vi "PWM FPGA Dephasing_no state machine2.vi"() -> ()   [LabVIEW 2013]
uses:
  <vilib>/eio/EIONode/EIONode.xnode
  <vilib>/rvi/eio/common/nirviEmuTemplateMethod_errors.vi
panel:
  out "Substract 2":i16
  out "Substract 1":i16
  out "Wait 2":i16
  out "Wait 1":i16
  in  "Remove Button":bool
  in  "Add Button":bool
  in  "Enable":bool
  in  "Direction":bool
  in  "Cluster":T1
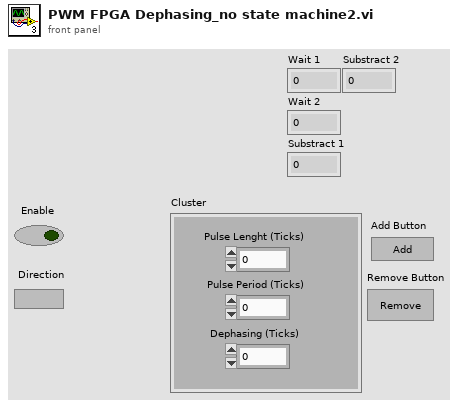
[diagram p1: front panel]
types:
  T1 = cluster{"Pulse Lenght (Ticks)":i16, "Pulse Period (Ticks)":i16, "Dephasing (Ticks)":i16}
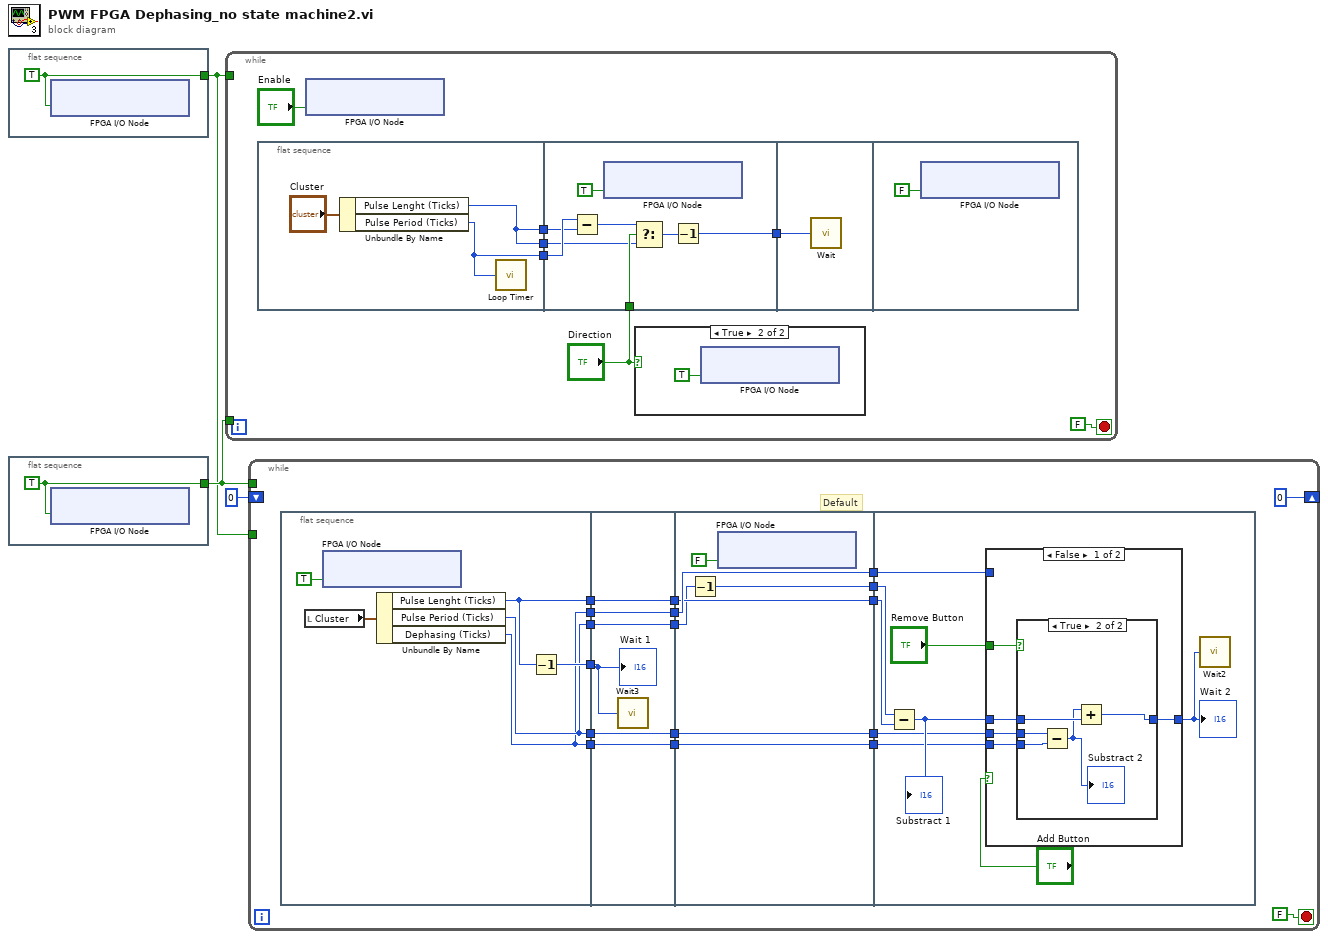
[diagram p0: block diagram]
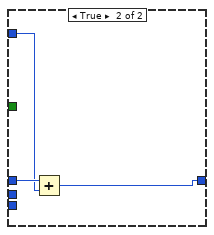
[diagram p3: hidden frame]
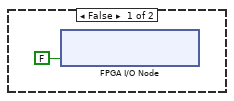
[diagram p4: hidden frame]
diagram:
  n1 = flat-sequence {
    tunnel: [w4] -> w1
    frame #0 {
      w4 = TRUE
      n2 = xnode "FPGA I/O Node"("ConnectorC/DIO3"=w4) -> ()  [unwired: 1 in, 1 out]
    }
  }
  n3 = flat-sequence {
    tunnel: [w5] -> w2
    frame #0 {
      w5 = TRUE
      n4 = xnode "FPGA I/O Node"("ConnectorC/DIO0"=w5) -> ()  [unwired: 1 in, 1 out]
    }
  }
  n5 = while {
    tunnel: w1 -> [_]
    tunnel: w2 -> [_]
    stop <- FALSE stop-if-true
    n6 = flat-sequence {
      tunnel: [w16] -> w12
      tunnel: [w17] -> w9
      tunnel: [w16] -> w8
      tunnel: w12 -> [w18]
      tunnel: [w24] -> w11
      tunnel: w9 -> [w22]
      tunnel: w8 -> [w21]
      tunnel: "Direction" -> [w20]
      tunnel: w11 -> [w26]
      frame #0 {
        n7 = Unbundle By Name("Cluster") -> ("Pulse Lenght (Ticks)"=w16:i16, "Pulse Period (Ticks)"=w17:i16)
        n8 = call "Loop Timer"("Count(Ticks)"=w17) -> ()  [unwired: 1 out]
      }
      frame #1 {
        n9 = Subtract(x=w22, y=w21) -> (x-y=w19:i16)
        n10 = xnode "FPGA I/O Node"("ConnectorC/DIO3"=TRUE ("ConnectorC/DIO7")) -> ()  [unwired: 1 in, 1 out]
        n11 = Select(t=w19, s=w20, f=w18) -> (s? t:f=w23:i16)
        n12 = Decrement(x=w23) -> (x-1=w24:i16)
      }
      frame #2 {
        n13 = call "Wait"("Count(Ticks)"=w26) -> ()  [unwired: 1 out]
      }
      frame #3 {
        n14 = xnode "FPGA I/O Node"("ConnectorC/DIO3"=FALSE ("ConnectorC/DIO7")) -> ()  [unwired: 1 in, 1 out]
      }
    }
    n15 = xnode "FPGA I/O Node"("ConnectorA/DIO0"="Enable") -> ()  [unwired: 1 in, 1 out]
    n16 = case shown="True" "Direction" {
      frame False {
        n17 = xnode "FPGA I/O Node"("ConnectorC/DIO7"=FALSE) -> ()  [unwired: 1 in, 1 out]
      }
      frame True {
        n18 = xnode "FPGA I/O Node"("ConnectorC/DIO7"=TRUE) -> ()  [unwired: 1 in, 1 out]
      }
    }
  }
  n19 = while {
    shift-right: [i16 0] -> _
    shift-left: i16 0 -> [_]
    tunnel: w2 -> [_]
    tunnel: w1 -> [_]
    stop <- FALSE stop-if-true
    # "Default"
    n20 = flat-sequence {
      tunnel: [w49] -> w43
      tunnel: [w47] -> w42
      tunnel: [w48] -> w37
      tunnel: [w46] -> w34
      tunnel: [w47] -> w31
      tunnel: [w46] -> w28
      tunnel: w43 -> [w57]
      tunnel: w42 -> [w56]
      tunnel: [w56] -> w41
      tunnel: [w55] -> w38
      tunnel: w37 -> [w55]
      tunnel: [w54] -> w35
      tunnel: w34 -> [w54]
      tunnel: [w53] -> w32
      tunnel: w31 -> [w53]
      tunnel: [w52] -> w29
      tunnel: w28 -> [w52]
      tunnel: w41 -> [w59]
      tunnel: [w58] -> w40
      tunnel: [w60] -> w39
      tunnel: w38 -> [w60]
      tunnel: [w63] -> w36
      tunnel: w35 -> [w63]
      tunnel: [w62] -> w33
      tunnel: w32 -> [w62]
      tunnel: [w61] -> w30
      tunnel: w29 -> [w61]
      tunnel: w40 -> [w71]
      tunnel: w39 -> [w70]
      tunnel: w36 -> [w67]
      tunnel: w33 -> [w66]
      tunnel: w30 -> [w65]
      frame #0 {
        n21 = local read "Cluster"() -> (w50:T1)
        n22 = xnode "FPGA I/O Node"("ConnectorC/DIO0"=TRUE ("ConnectorC/DIO7")) -> ()  [unwired: 1 in, 1 out]
        n23 = Unbundle By Name(w50) -> ("Pulse Lenght (Ticks)"=w48:i16, "Pulse Period (Ticks)"=w47:i16, "Dephasing (Ticks)"=w46:i16)
        n24 = Decrement(x=w48) -> (x-1=w49:i16)
      }
      frame #1 {
        n25 = call "Wait3"("Count(Ticks)"=w57) -> ()  [unwired: 1 out]
        "Wait 1" <- w57
      }
      frame #2 {
        n26 = Decrement(x=w59) -> (x-1=w58:i16)
        n27 = xnode "FPGA I/O Node"("ConnectorC/DIO0"=FALSE ("ConnectorC/DIO7")) -> ()  [unwired: 1 in, 1 out]
      }
      frame #3 {
        n28 = Subtract(x=w71, y=w70) -> (x-y=w69:i16)
        "Substract 1" <- w69
        n29 = case shown="False" "Add Button" {
          tunnel: "Remove Button" -> [w78 _]
          tunnel: w69 -> [w77 w87]
          tunnel: [w76 w85] -> w68
          tunnel: w67 -> [_ w86]
          tunnel: w66 -> [w75 _]
          tunnel: w65 -> [w74 _]
          frame False {
            n30 = case shown="True" w78 {
              tunnel: [w79 w81] -> w76
              tunnel: w77 -> [w79 w82]
              tunnel: w75 -> [_ w84]
              tunnel: w74 -> [_ w83]
              frame False {
              }
              frame True {
                n31 = Subtract(x=w84, y=w83) -> (x-y=w80:i16)
                "Substract 2" <- w80
                n32 = Add(x=w80, y=w82) -> (x+y=w81:i16)
              }
            }
          }
          frame True {
            n33 = Add(x=w87, y=w86) -> (x+y=w85:i16)
          }
        }
        "Wait 2" <- w68
        n34 = call "Wait2"("Count(Ticks)"=w68) -> ()  [unwired: 1 out]
      }
    }
  }
